vi "Update_all.vi"(7 "# axis":i32, 8 "error in (no error)":errorcluster, 11 "VISA resource name":refnum<visa-resource-name>) -> (0 "error out":errorcluster, 1 "Moving":bool, 2 "Currrent postion":dbl[](array[numeric]), 3 "tickcount_pos":u32, 5 "MotorDisabled":bool)   [LabVIEW 2012, in "ESP300.lvlib"]
doc: "Performs an instrument error query before terminating the software connection to the instrument."
uses:
  <instrlib>/ESP300/ESP300.lvlib
  <instrlib>/ESP300/Public/Position_ESP300.vi
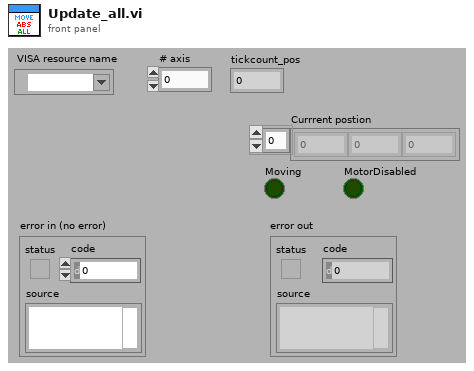
[diagram p1: front panel]
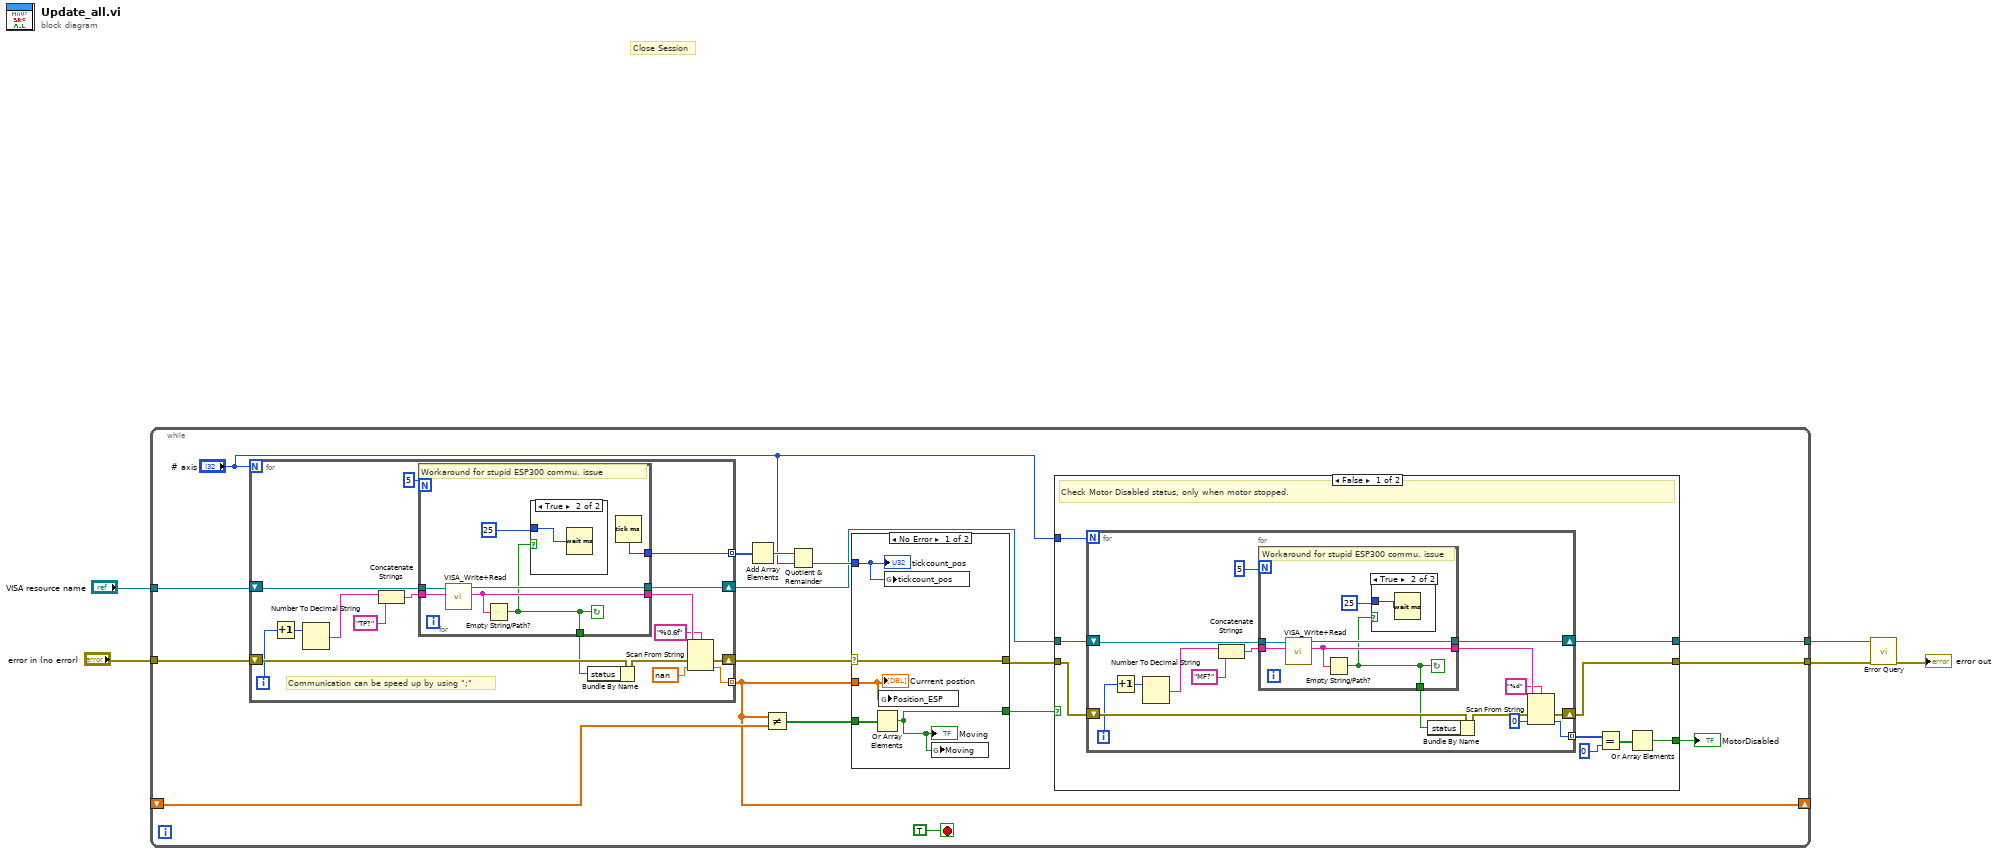
[diagram p0: block diagram]
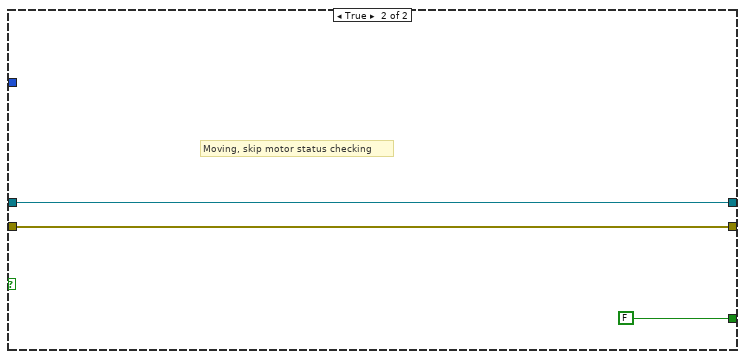
[diagram p3: hidden frame]
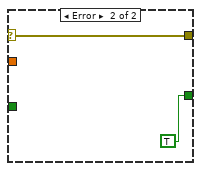
[diagram p4: hidden frame]
diagram:
  # "Close Session"
  n1 = while {
    tunnel: "error in (no error)" -> [w22]
    tunnel: "VISA resource name" -> [w19]
    shift-right: [w15] -> _
    shift-left: _ -> [w18]
    tunnel: [w7] -> w1
    tunnel: [w6] -> w2
    stop <- TRUE stop-if-true
    n2 = for {
      N: "# axis" -> [_]
      tunnel: [w75] -> w15 mode=indexing
      shift-right: [w76] -> w14
      shift-left: w22 -> [w79]
      tunnel: [w69] -> w21 mode=indexing
      shift-right: [w68] -> w10
      shift-left: w19 -> [w77]
      i -> [w74]
      # "Communication can be speed up by using \";\""
      n3 = Increment(x=w74) -> (x+1=w70:i32)
      n4 = Number To Decimal String(number=w70) -> (decimal integer string=w71:string)  [unwired: 1 in]
      n5 = Concatenate Strings(w71, "TP?" ("string")) -> (w73:string)
      n6 = for {
        N: 5 -> [_]
        tunnel: [w84] -> w81
        tunnel: w77 -> [w88]
        tunnel: w73 -> [w87]
        tunnel: [w86] -> w69
        tunnel: [w85] -> w68
        tunnel: [w82] -> w65
        stop <- w82 continue-if-true
        # "Workaround for stupid ESP300 commu. issue"
        n7 = call <instrlib>:"VISA_Write+Read.vi"("Write Buffer"=w87, "VISA resource name"=w88) -> ("readout"=w84:string, "VISA resource name out"=w85:refnum<visa-resource-name>)  [unwired: 7 in, 1 out]
        n8 = Empty String/Path?(string/path=w84) -> (empty?=w82:bool)
        n9 = case shown="True" w82 {
          tunnel: u32 25 ("milliseconds to wait") -> [_ w89]
          frame False {
          }
          frame True {
            n10 = Wait (ms)(milliseconds to wait=w89) -> ()  [unwired: 1 out]
          }
        }
        n11 = Tick Count (ms)() -> (millisecond timer value=w86:u32)
      }
      n12 = Bundle By Name(cluster=w79, "status"=w65) -> (w66:errorcluster)
      n13 = Scan From String(format string="%0.6f", input string=w81, error in=w66, default 1=nan ("default value 1")) -> (error out=w76:errorcluster, output 1=w75:dbl)  [unwired: 1 in, 2 out]
    }
    n14 = Add Array Elements(numeric array=w21) -> (sum=w20:u32)
    n15 = Not Equal?(x=w15, y=w18) -> (x != y?=w13:bool[])
    n16 = Quotient & Remainder(x=w20, y="# axis") -> (floor(x/y)=w16:u32)  [unwired: 1 out]
    n17 = case shown="No Error" w14 {
      selector: w14 -> [w60 w64]
      tunnel: w16 -> [w62 _]
      tunnel: w15 -> [w61 _]
      tunnel: [w60 w64] -> w8
      tunnel: w13 -> [w59 _]
      tunnel: [w58 TRUE] -> w12
      frame No Error {
        n18 = Or Array Elements(Boolean array=w59) -> (logical OR=w58:bool)
        "Moving" <- w58
        n19 = global write "Position_ESP300.vi" "Position_ESP"(w61) -> ()
        n20 = global write "Position_ESP300.vi" "tickcount_pos"(w62) -> ()
        n21 = global write "Position_ESP300.vi" "Moving"(w58) -> ()
        "Currrent postion" <- w61
        "tickcount_pos" <- w62
      }
      frame Error {
      }
    }
    n22 = case shown="False" w12 {
      tunnel: [w27 FALSE] -> w11
      tunnel: w10 -> [w26 w56]
      tunnel: "# axis" -> [w31 _]
      tunnel: [w25 w56] -> w7
      tunnel: [w24 w55] -> w6
      tunnel: w8 -> [w23 w55]
      frame False {
        # "Check Motor Disabled status, only when motor stopped."
        n23 = for {
          N: w31 -> [_]
          tunnel: [w42] -> w30 mode=indexing
          shift-right: [w43] -> w24
          shift-left: w23 -> [w45]
          shift-right: [w36] -> w25
          shift-left: w26 -> [w44]
          i -> [w41]
          n24 = Increment(x=w41) -> (x+1=w37:i32)
          n25 = Number To Decimal String(number=w37) -> (decimal integer string=w38:string)  [unwired: 1 in]
          n26 = Concatenate Strings(w38, "MF?" ("string")) -> (w40:string)
          n27 = for {
            N: 5 -> [_]
            tunnel: [w50] -> w47
            tunnel: w44 -> [w53]
            tunnel: w40 -> [w52]
            tunnel: [w51] -> w36
            tunnel: [w48] -> w33
            stop <- w48 continue-if-true
            # "Workaround for stupid ESP300 commu. issue"
            n28 = call <instrlib>:"VISA_Write+Read.vi"("Write Buffer"=w52, "VISA resource name"=w53) -> ("readout"=w50:string, "VISA resource name out"=w51:refnum<visa-resource-name>)  [unwired: 7 in, 1 out]
            n29 = Empty String/Path?(string/path=w50) -> (empty?=w48:bool)
            n30 = case shown="True" w48 {
              tunnel: u32 25 ("milliseconds to wait") -> [_ w54]
              frame False {
              }
              frame True {
                n31 = Wait (ms)(milliseconds to wait=w54) -> ()  [unwired: 1 out]
              }
            }
          }
          n32 = Bundle By Name(cluster=w45, "status"=w33) -> (w34:errorcluster)
          n33 = Scan From String(format string="%d", input string=w47, error in=w34, default 1=0 ("default value 1")) -> (error out=w43:errorcluster, output 1=w42:i32)  [unwired: 1 in, 2 out]
        }
        n34 = Equal?(x=w30, y=0 ("default value 1")) -> (x = y?=w28:bool[])
        n35 = Or Array Elements(Boolean array=w28) -> (logical OR=w27:bool)
      }
      frame True {
        # "Moving, skip motor status checking"
      }
    }
    "MotorDisabled" <- w11
  }
  n36 = call <instrlib>:"Error Query.vi"("error in (no error)"=w2, "VISA resource name"=w1) -> ("error out"=→"error out":errorcluster)  [unwired: 6 in, 3 out]
